vi "ConvertBoundingRect2fourpoints.vi"(8 "Error In":errorcluster, 11 "Bounding Box":cluster{"x":sgl, "y":sgl}[](array[cluster])) -> (0 "Error Out":errorcluster, 3 "Array":i32[](array[numeric]))   [LabVIEW 2013]
panel:
  # "output"
  # "input"
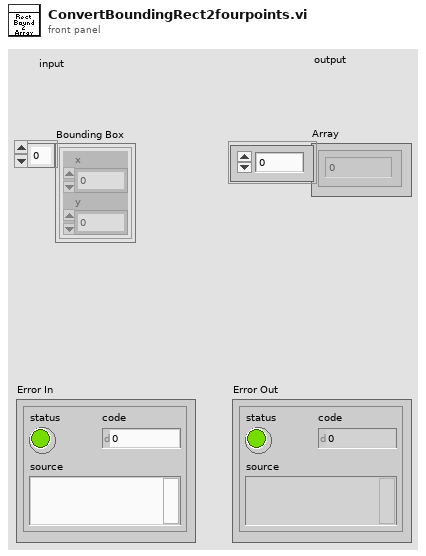
[diagram p1: front panel]
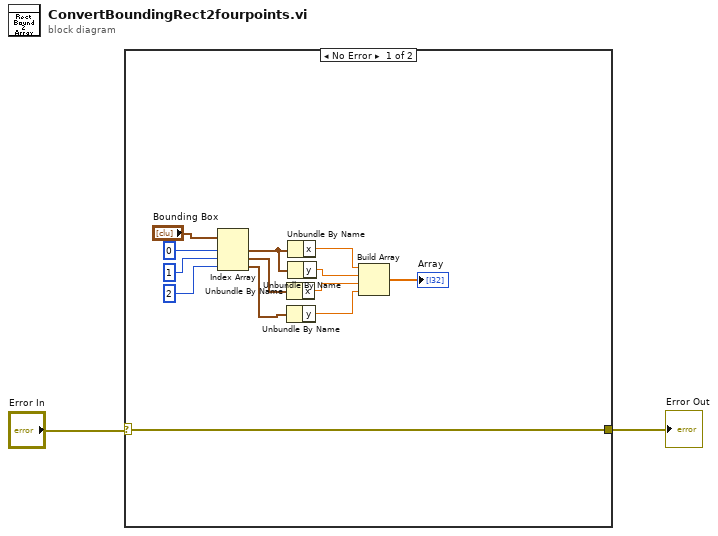
[diagram p0: block diagram]
diagram:
  n1 = case shown="No Error" "Error In" {
    selector: "Error In" -> [w15 w16]
    tunnel: [w15 w16] -> w1
    frame No Error {
      n2 = Index Array(array="Bounding Box", index #1=0 ("index"), index #2=1 ("index"), index #3=2 ("index")) -> (element #1=w3:cluster{"x":sgl, "y":sgl}, element #2=w5:cluster{"x":sgl, "y":sgl}, element #3=w4:cluster{"x":sgl, "y":sgl})
      n3 = Unbundle By Name(w5) -> ("x"=w8:sgl)
      n4 = Unbundle By Name(w4) -> ("y"=w7:sgl)
      n5 = Unbundle By Name(w3) -> ("x"=w10:sgl)
      n6 = Unbundle By Name(w3) -> ("y"=w9:sgl)
      n7 = Build Array(w10, w9, w8, w7) -> (→"Array":sgl[])
    }
    frame Error {
    }
  }
  "Error Out" <- w1
